vi "Notifier_Driver.vi"(0 "Notification":bool, 2 "Notifier_Name":string, 11 "Error_In":errorcluster, 13 "Notifier_Operation_Select":T1=enum."Get_Notification_Status") -> (4 "Latest_Notification":bool, 15 "Error_Out":errorcluster)   [LabVIEW 2021]
doc: "Used to Create, Send, Receive and release the notifier."
uses:
  Controls/Notifier_Operation_Select.ctl
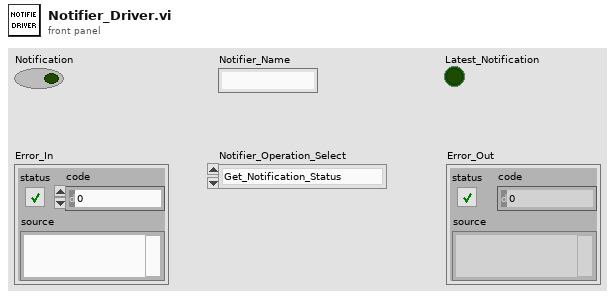
[diagram p1: front panel]
types:
  T1 = typedef "Notifier_Operation_Select.ctl" = enum16{"Obtain_Notification", "Send_Notification", "Get_Notification_Status", "Release_Notification"}
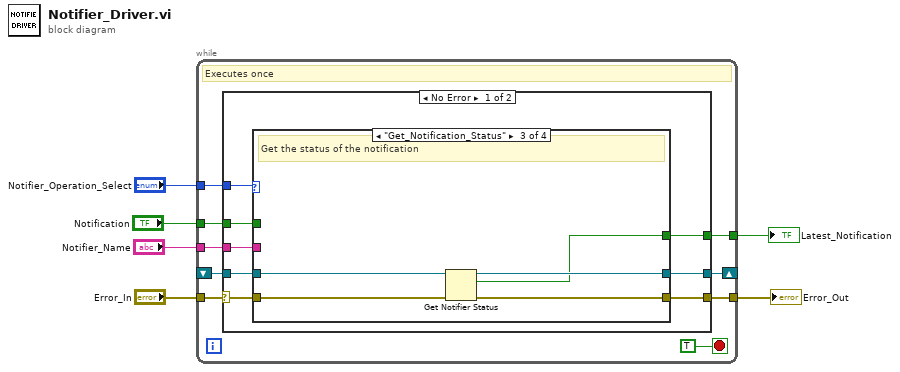
[diagram p0: block diagram]
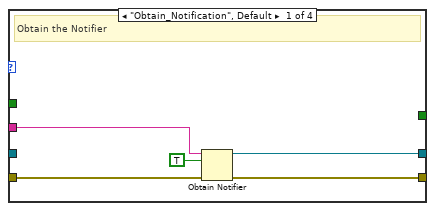
[diagram p2: hidden frame]
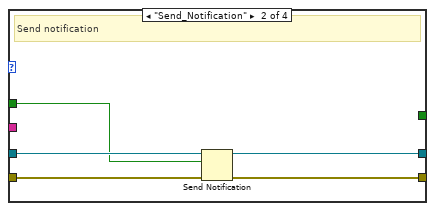
[diagram p3: hidden frame]
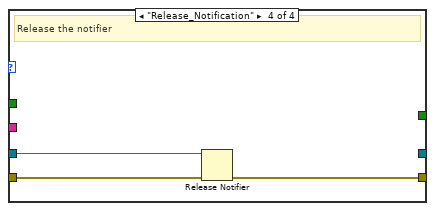
[diagram p4: hidden frame]
diagram:
  n1 = while {
    tunnel: "Error_In" -> [w15]
    tunnel: [w13] -> w5
    tunnel: "Notifier_Name" -> [w12]
    shift-right: [w11] -> _
    shift-left: _ -> [w10]
    tunnel: "Notification" -> [w9]
    tunnel: "Notifier_Operation_Select" -> [w8]
    tunnel: [w7] -> w1
    stop <- TRUE stop-if-true
    # "Executes once"
    n2 = case shown="No Error" w15 {
      selector: w15 -> [w22 w43]
      tunnel: [w23 w43] -> w13
      tunnel: w12 -> [w21 _]
      tunnel: [w20 w42] -> w11
      tunnel: w10 -> [w19 w42]
      tunnel: w9 -> [w18 _]
      tunnel: w8 -> [w17 _]
      tunnel: [w16 _] -> w7
      frame No Error {
        n3 = case shown="\"Get_Notification_Status\"" w17 {
          tunnel: [w27 w32 w37 w40] -> w23
          tunnel: w22 -> [w28 w33 w38 w41]
          tunnel: w21 -> [w25 _ _ _]
          tunnel: [w24 w29 w35 _] -> w20
          tunnel: w19 -> [_ w31 w36 w39]
          tunnel: w18 -> [_ w30 _ _]
          tunnel: [_ _ w34 _] -> w16
          frame "Obtain_Notification", Default {
            # "Obtain the Notifier"
            n4 = Obtain Notifier(name (unnamed)=w25, notification data type=TRUE, error in (no error)=w28) -> (notifier out=w24:refnum<notifier>, error out=w27:errorcluster)  [unwired: 1 in, 1 out]
          }
          frame "Send_Notification" {
            # "Send notification"
            n5 = Send Notification(notification=w30, notifier=w31, error in (no error)=w33) -> (notifier out=w29:refnum<notifier>, error out=w32:errorcluster)
          }
          frame "Get_Notification_Status" {
            # "Get the status of the notification"
            n6 = Get Notifier Status(notifier=w36, error in (no error)=w38) -> (notifier out=w35:refnum<notifier>, current notification=w34:bool, error out=w37:errorcluster)  [unwired: 2 out]
          }
          frame "Release_Notification" {
            # "Release the notifier"
            n7 = Release Notifier(notifier=w39, error in (no error)=w41) -> (error out=w40:errorcluster)  [unwired: 1 in, 2 out]
          }
        }
      }
      frame Error {
      }
    }
  }
  "Error_Out" <- w5
  "Latest_Notification" <- w1
